vi "KE622x -- Set Meas Elements.vi"(0 "Resource In":refnum<visa-resource-name>, 1 "Check For SCPI Errors? (T)":bool=TRUE, 7 "Meas Elements To Return":T1={"Timstamp?"=TRUE, "Reading Num?"=TRUE, "Source Value?"=FALSE, "Compliance?"=FALSE, "Average Voltage?"=FALSE}, 11 "error in (no error)":errorcluster) -> (4 "Resource Out (dupl)":refnum<visa-resource-name>, 15 "error out":errorcluster)   [LabVIEW 2019, in "Keithley 622x.lvlib"]
doc: "Allows the user to specify which data fields will be returned when the trace buffer is read. Note that all fields are _always_ stored -- this VI just lets the user specify which ones to return."
uses:
  Keithley 622x.lvlib
  Typedefs/KE622x -- Optional Meas Elements.ctl
panel:
  # "*** NOTE:  \"Average Voltage\"\nis only available for Differential\nConductance measurements."
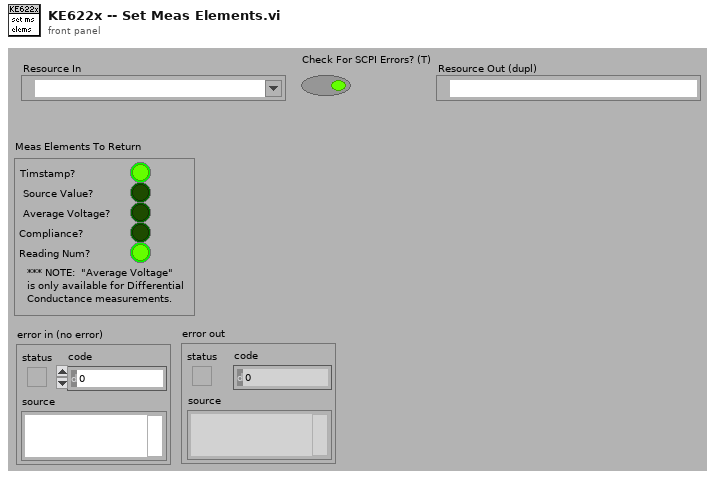
[diagram p1: front panel]
types:
  T1 = typedef "Keithley 622x.lvlib/KE622x -- Optional Meas Elements.ctl" = cluster{"Timstamp?":bool, "Reading Num?":bool, "Source Value?":bool, "Compliance?":bool, "Average Voltage?":bool}
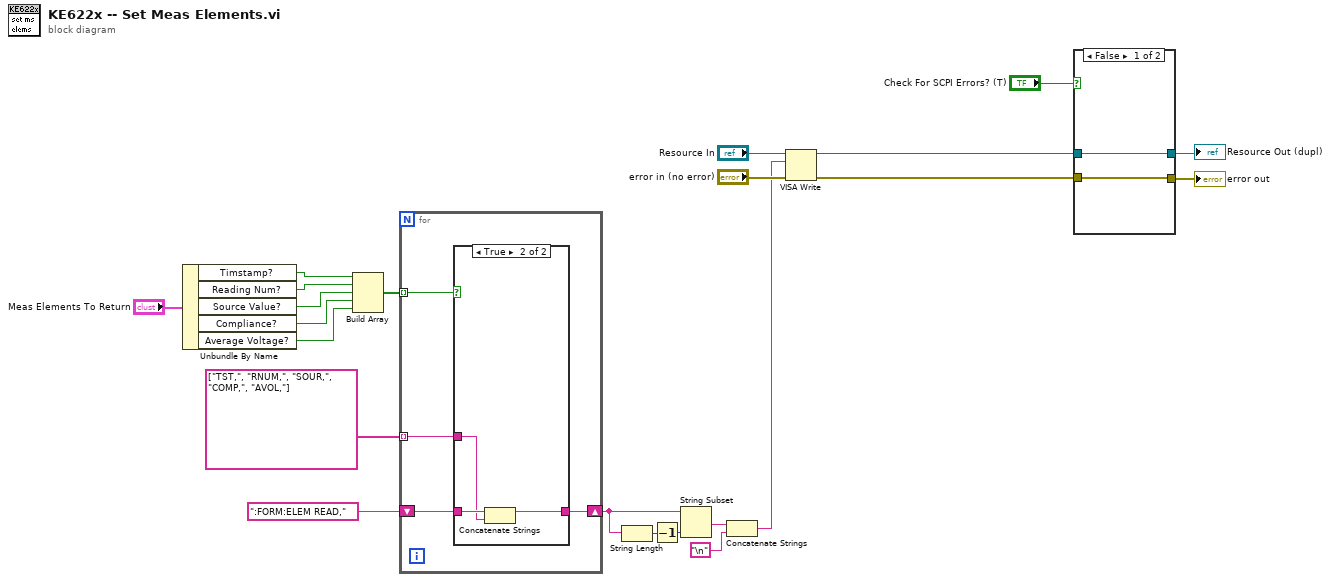
[diagram p0: block diagram]
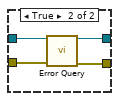
[diagram p3: hidden frame]
diagram:
  n1 = Unbundle By Name("Meas Elements To Return") -> ("Timstamp?"=w14:bool, "Reading Num?"=w13:bool, "Source Value?"=w12:bool, "Compliance?"=w11:bool, "Average Voltage?"=w10:bool)
  n2 = Build Array(w14, w13, w12, w11, w10) -> (w9:bool[])
  n3 = for {
    tunnel: w9 -> [w26] mode=indexing
    tunnel: string[] ["TST,", "RNUM,", "SOUR,", "COMP,", "AVOL,"] -> [w25] mode=indexing
    shift-right: [w23] -> w4
    shift-left: ":FORM:ELEM READ," ("format string") -> [w24]
    n4 = case shown="True" w26 {
      tunnel: w25 -> [_ w29]
      tunnel: w24 -> [w27 w30]
      tunnel: [w27 w28] -> w23
      frame False {
      }
      frame True {
        n5 = Concatenate Strings(w30, w29) -> (w28:string)
      }
    }
  }
  n6 = String Length(string=w4) -> (length=w6:i32)
  n7 = Decrement(x=w6) -> (x-1=w5:i32)
  n8 = String Subset(string=w4, length (rest)=w5) -> (substring=w3:string)  [unwired: 1 in]
  n9 = Concatenate Strings(w3, "\n") -> (w1:string)
  n10 = VISA Write(VISA resource name="Resource In", write buffer=w1, error in (no error)="error in (no error)") -> (VISA resource name out=w19:refnum<visa-resource-name>, error out=w18:errorcluster)  [unwired: 1 out]
  n11 = case shown="False" "Check For SCPI Errors? (T)" {
    tunnel: w19 -> [w32 w36]
    tunnel: w18 -> [w31 w35]
    tunnel: [w31 w34] -> w16
    tunnel: [w32 w33] -> w17
    frame False {
    }
    frame True {
      n12 = call "Error Query.vi"("VISA Resource In"=w36, "error in (no error)"=w35) -> ("VISA Resource Out (dupl)"=w33:refnum<visa-resource-name>, "error out"=w34:errorcluster)  [unwired: 10 in, 2 out]
    }
  }
  "Resource Out (dupl)" <- w17
  "error out" <- w16
